vi "CD Read Engine_Parse Message_Update Tx SA RT Timestamp channel for RT to RT Frame.vi"(7 "record in":T10 {"type" format="%04x"; "activity" format="%04x"; "error" format="%04x"; "cwd1" format="%04x"; "cwd2" format="%04x"; "swd1" format="%04x"; "swd2" format="%04x"; "data" format="%04x"}, 8 "error in (no error)":errorcluster, 10 "Frame Drescriptors":T1[](array[typedef]) {"RT"."Status Channel Ref" format="%.0x"; "RT"."Words Block Data Refs"."Data Reference" format="%.0x"; "RT"."Timestamp Channel Data Reference" format="%.0x"; "BC"."Status Channel Refs" format="%.0x"; "BC"."Words Block Data Refs"."Data Reference" format="%.0x"; "BC"."Timestamp Channel Data Reference" format="%.0x"}, 11 "Timestamp (s)":dbl) -> (0 "error out":errorcluster)   [LabVIEW 2017, in "Ballard MIL-1553 Engine.lvlib"]
doc: "This VI is used to update the Timestamp Channel of the Tx RT for RT 2 RT frames (Broadcast or not)."
uses:
  Ballard MIL-1553 Engine.lvlib
  <instrlib>/BTICardLib/Public/Controls/1553 Record.ctl
  Controls/RT Inline Frame Descriptor.ctl
  Controls/RT Inline Frame Descriptor_BC.ctl
  <vilib>/NI Veristand/Custom Device API/Data Reference.ctl
  <vilib>/NI Veristand/Custom Device API/Block Data Reference.ctl
  <vilib>/NI Veristand/Custom Device API/Custom Device Item Ref.ctl
  Controls/RT Inline Frame Descriptor_RT.ctl
  Shared/Controls and Global/RT CWD2.ctl
  Shared/Controls and Global/RT CWD1.ctl
  Shared/Controls and Global/RT messageType.ctl
  <vilib>/NI Veristand/Custom Device API/Global Data Refs.vi
  <vilib>/NI VeriStand/Custom Device API/Custom Device API.lvlib
  <vilib>/NI VeriStand/Custom Device Tools/Custom Device Utility Library/Custom Device Utility Library.lvlib
  <instrlib>/BTICardLib/BTICardLV.lvlib
  Shared/Ballard 1553 Shared.lvlib
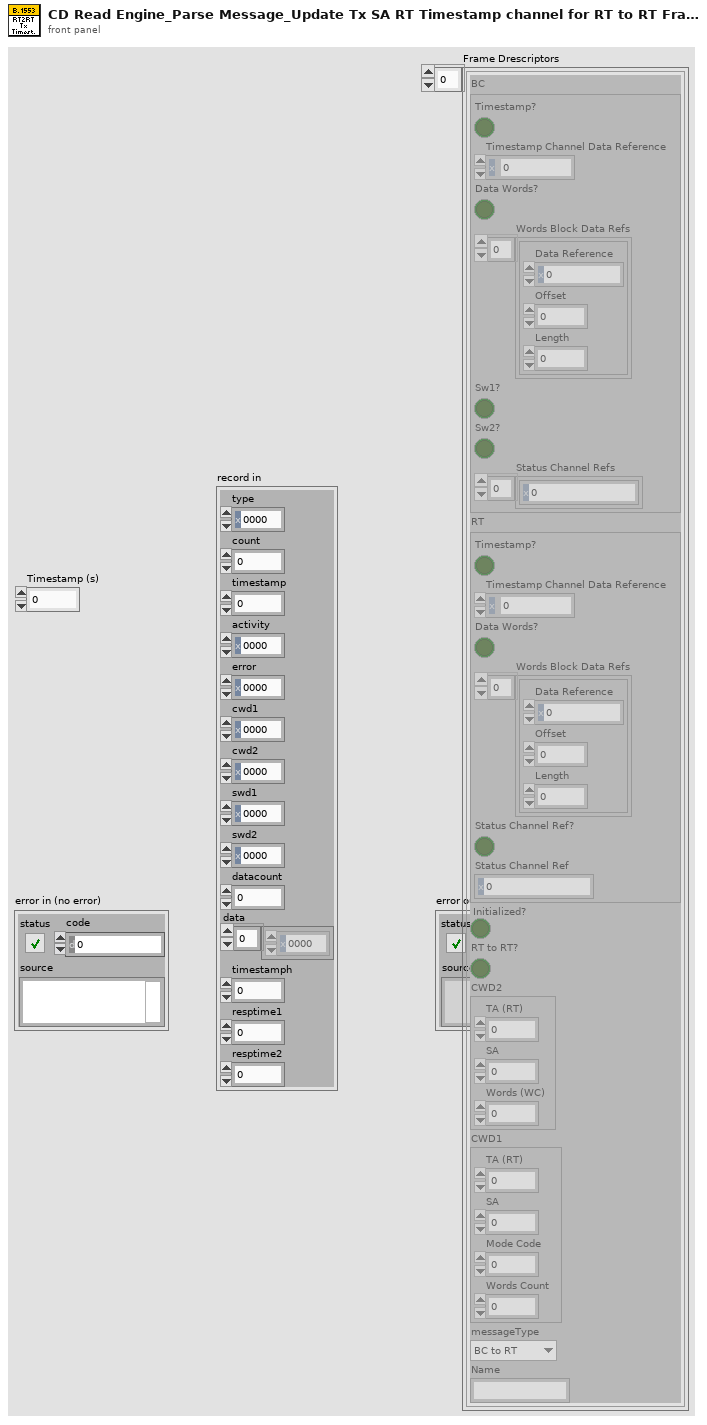
[diagram p1: front panel]
types:
  T1 = typedef "Ballard MIL-1553 Engine.lvlib/RT Inline Frame Descriptor.ctl" = cluster{"BC":T2, "RT":T6, "Initialized?":bool, "RT to RT?":bool, "CWD2":T7, "CWD1":T8, "messageType":T9, "Name":string}
  T2 = typedef "Ballard MIL-1553 Engine.lvlib/RT Inline Frame Descriptor_BC.ctl" = cluster{"Timestamp?":bool, "Timestamp Channel Data Reference":T3, "Data Words?":bool, "Words Block Data Refs":T4[], "Sw1?":bool, "Sw2?":bool, "Status Channel Refs":T5[]}
  T3 = typedef "Custom Device API.lvlib/Data Reference.ctl" = i32
  T4 = typedef "Custom Device API.lvlib/Block Data Reference.ctl" = cluster{"Data Reference":T3, "Offset":u64, "Length":u64}
  T5 = typedef "Custom Device API.lvlib/Custom Device Item Ref.ctl" = u64
  T6 = typedef "Ballard MIL-1553 Engine.lvlib/RT Inline Frame Descriptor_RT.ctl" = cluster{"Timestamp?":bool, "Timestamp Channel Data Reference":T3, "Data Words?":bool, "Words Block Data Refs":T4[], "Status Channel Ref?":bool, "Status Channel Ref":T5}
  T7 = typedef "Ballard 1553 Shared.lvlib/RT CWD2.ctl" = cluster{"TA (RT)":i8, "SA":i8, "Words (WC)":i8}
  T8 = typedef "Ballard 1553 Shared.lvlib/RT CWD1.ctl" = cluster{"TA (RT)":i8, "SA":i8, "Mode Code":i8, "Words Count":i8}
  T9 = typedef "Ballard 1553 Shared.lvlib/RT messageType.ctl" = enum16{"BC to RT", "RT to BC", "RT to RT", "MC (Rx)", "MC (Tx)"}
  T10 = typedef "BTICardLV.lvlib/1553 Record.ctl" = cluster{"type":u16, "count":u16, "timestamp":u32, "activity":u16, "error":u16, "cwd1":u16, "cwd2":u16, "swd1":u16, "swd2":u16, "datacount":u16, "data":u16[], "timestamph":u32, "resptime1":u16, "resptime2":u16}
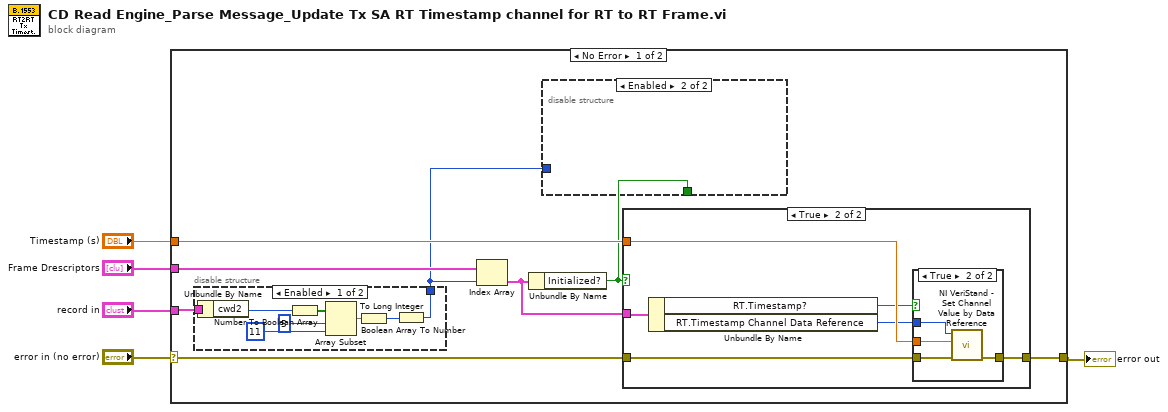
[diagram p0: block diagram]
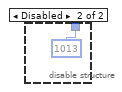
[diagram p2: hidden frame]
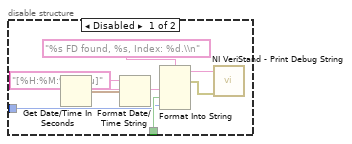
[diagram p3: hidden frame]
diagram:
  n1 = case shown="No Error" "error in (no error)" {
    selector: "error in (no error)" -> [w11 w43]
    tunnel: [w10 w43] -> w4
    tunnel: "record in" -> [w13 _]
    tunnel: "Frame Drescriptors" -> [w12 _]
    tunnel: "Timestamp (s)" -> [w9 _]
    frame No Error {
      n2 = disable-structure shown="Enabled" {
        disable-tunnel: w13 -> [w21 _]
        disable-tunnel: [w14 1013] -> w6
        frame Enabled {
          n3 = Unbundle By Name(w21) -> ("cwd2"=w15:u16)
          n4 = Number To Boolean Array(number=w15) -> (Boolean array=w19:bool[])
          n5 = Array Subset(array=w19, index=5, length=11) -> (w17:bool[])
          n6 = Boolean Array To Number(Boolean array=w17) -> (number=w16:u32)
          n7 = To Long Integer(number=w16) -> (32bit integer=w14:i32)
        }
        frame Disabled {
        }
      }
      n8 = Index Array(array=w12, index=w6) -> (element=w8:T1)
      n9 = Unbundle By Name(w8) -> ("Initialized?"=w7:bool)
      n10 = disable-structure shown="Enabled" {
        disable-tunnel: w7 -> [w24 _]
        disable-tunnel: w6 -> [w23 _]
        frame Disabled {
          n11 = Get Date/Time In Seconds() -> (seconds since 1Jan1904=w30:timestamp)
          n12 = Format Date/Time String(time format string (%c)="[%H:%M:%S%3u]", seconds (now)=w30) -> (date/time string=w29:string)  [unwired: 1 in]
          n13 = Format Into String(format string="%s FD found, %s, Index: %d.\\n", w29, w24, w23) -> (resulting string=w25:string, error out=w26:errorcluster)  [unwired: 2 in]
          n14 = call <vilib>:"NI VeriStand - Print Debug String.vi"("error in (no error)"=w26, "Message"=w25) -> ()  [unwired: 9 in, 1 out]
        }
        frame Enabled {
        }
      }
      n15 = case shown="True" w7 {
        tunnel: w11 -> [w31 w36]
        tunnel: [w31 w33] -> w10
        tunnel: w9 -> [_ w35]
        tunnel: w8 -> [_ w37]
        frame False {
        }
        frame True {
          n16 = Unbundle By Name(w37) -> ("RT.Timestamp?"=w34:bool, "RT.Timestamp Channel Data Reference"=w32:T3)
          n17 = case shown="True" w34 {
            tunnel: w35 -> [_ w42]
            tunnel: w36 -> [w38 w41]
            tunnel: [w38 w40] -> w33
            tunnel: w32 -> [_ w39]
            frame False {
            }
            frame True {
              n18 = call <vilib>:"NI VeriStand - Set Channel Value by Data Reference.vi"("error in (no error)"=w41, "Value"=w42, "Data Reference in"=w39) -> ("error out"=w40:errorcluster)  [unwired: 8 in]
            }
          }
        }
      }
    }
    frame Error {
    }
  }
  "error out" <- w4
